vi "ConvertItemListToSenseFormatElements.vi"(11 "Item List":string) -> (3 "Sense Format Elements":T1[](array[typedef]))   [LabVIEW 2009, in "Keithley-6482-Visa.lvlib"]
uses:
  <instrlib>/Keithley-6482-Visa9.0/Keithley-6482-Visa.lvlib
  <instrlib>/Keithley-6482-Visa9.0/Public/Controls/SenseFormatElement.ctl
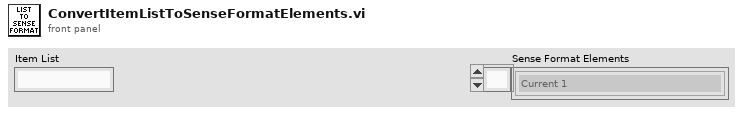
[diagram p1: front panel]
types:
  T1 = typedef "Keithley-6482-Visa.lvlib/SenseFormatElement.ctl" = enum16{"Current 1", "Current 2", "Time", "Status"}
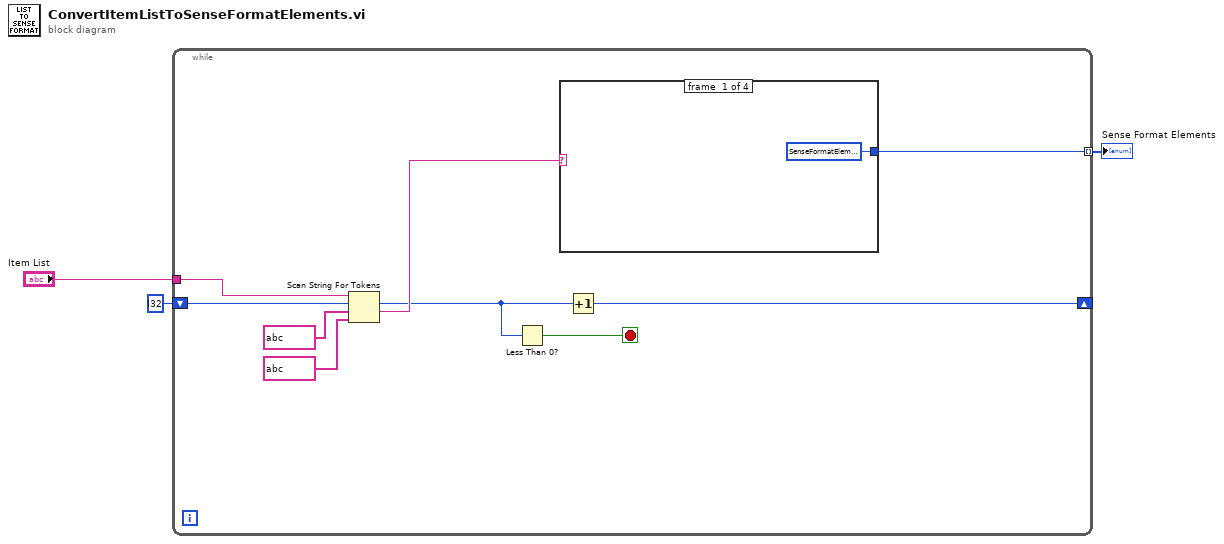
[diagram p0: block diagram]
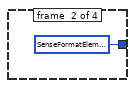
[diagram p2: hidden frame]
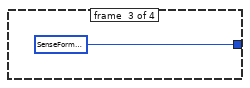
[diagram p3: hidden frame]
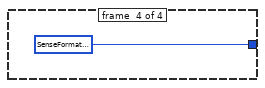
[diagram p4: hidden frame]
diagram:
  n1 = while {
    shift-right: [w4] -> _
    shift-left: i32 ? ("offset past token") -> [w12]
    tunnel: [w10] -> w2 mode=indexing
    tunnel: "Item List" -> [w7]
    stop <- w6 stop-if-true
    n2 = Scan String For Tokens(6:string[] ? ("delimiters (\\s,\\t,\\r,\\n)"), 7:string[] ? ("delimiters (\\s,\\t,\\r,\\n)"), 8:w12, 9:w7) -> (1:w11:string, 2:w5:i32)  [unwired: 2 in, 2 out]
    n3 = Less Than 0?(x=w5) -> (x < 0?=w6:bool)
    n4 = case shown="\"CURR2\"" w11 {
      tunnel: [T1 ? ("Format Sense Element") T1 ? ("Format Sense Element") T1 ? ("Format Sense Element") T1 ? ("Format Sense Element")] -> w10
      frame #0 {
      }
      frame #1 {
      }
      frame #2 {
      }
      frame #3 {
      }
    }
    n5 = Increment(x=w5) -> (x+1=w4:i32)
  }
  "Sense Format Elements" <- w2
